vi "Start-Scope.vi"(0 "VISA resource name":refnum<visa-resource-name>="Scope", 1 "Vertical Range (10.0 V)":dbl=10.0, 3 "Position (0.0 s)":dbl, 4 "Acquisition Type (0:Sample)":u16(ring)=3 items=["Sample", "Peak Detect", "Hi Res", "Average", "Envelope", "WfmDB"], 5 "Signal Channel":u16(ring)=1 format="%#_5f" items=["Channel 1", "Channel 2", "Channel 3", "Channel 4", "Math 1", "Math 2", "Math 3", "Math 4", "Reference 1", "Reference 2", "Reference 3", "Reference 4"], 6 "Average Waveforms (10)":i32=300, 9 "Trigger Channel":u16(ring) format="%#_5f" items=["Channel 1", "Channel 2", "Channel 3", "Channel 4", "Math 1", "Math 2", "Math 3", "Math 4", "Reference 1", "Reference 2", "Reference 3", "Reference 4"], 11 "Input Impedance (0: 1M ohm)":u16(ring)=1 items=["1M", "50"], 12 "Record Length (10000)":u32=10000 caption="Record Length (10000s)", 13 "Trigger Level (0.0V)":dbl=1.0) -> (2 "Average Waveforms (10) Out":i32=300, 8 "error out":errorcluster, 10 "Timebase":u32, 14 "VISA resource name out":refnum<visa-resource-name>, 15 "Signal Channel \nOut":u16(ring)=1 caption="Signal Channel" format="%#_5f" items=["Channel 1", "Channel 2", "Channel 3", "Channel 4", "Math 1", "Math 2", "Math 3", "Math 4", "Reference 1", "Reference 2", "Reference 3", "Reference 4"])   [LabVIEW 2018]
uses:
  <instrlib>/Tektronix 7000 Series/Public/Configure/Configure Trigger (Edge).vi
  <instrlib>/Tektronix 7000 Series/Tektronix 7000 Series.lvlib
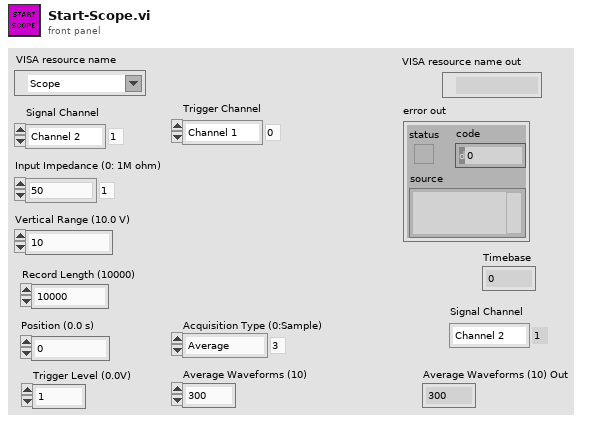
[diagram p1: front panel]
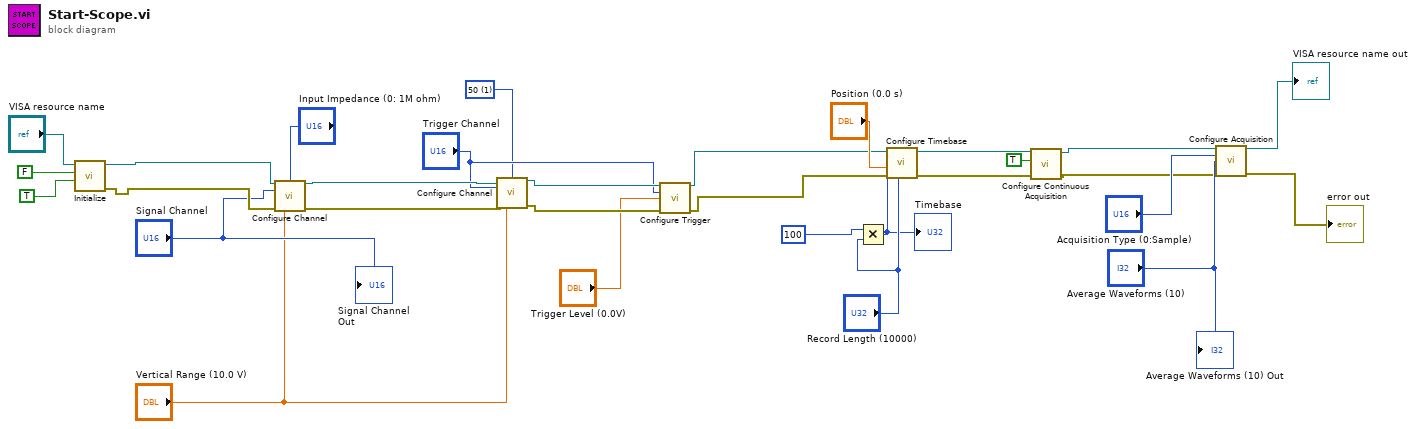
[diagram p0: block diagram]
diagram:
  w2 = u16 1 items=["1M", "50"] ("Input Impedance (0: 1M ohm)")
  n1 = call <instrlib>:"Initialize.vi"("Reset? ( Yes)"=TRUE, "ID Query? ( Yes)"=FALSE, "VISA resource name"="VISA resource name") -> ("error out"=w14:errorcluster, "VISA resource name out"=w15:refnum<visa-resource-name>)  [unwired: 7 in]
  n2 = call <instrlib>:"Configure Channel.vi"("VISA resource name"=w15, "Input Impedance (0: 1M ohm)"="Input Impedance (0: 1M ohm)", "Channel (0: Channel 1)"="Signal Channel", "error in (no error)"=w14, "Vertical Range (10.0 V)"="Vertical Range (10.0 V)") -> ("VISA resource name out"=w27:refnum<visa-resource-name>, "error out"=w26:errorcluster)  [unwired: 9 in]
  n3 = call <instrlib>:"Configure Channel.vi"("VISA resource name"=w27, "Input Impedance (0: 1M ohm)"=w2, "Channel (0: Channel 1)"="Trigger Channel", "error in (no error)"=w26, "Vertical Range (10.0 V)"="Vertical Range (10.0 V)") -> ("VISA resource name out"=w25:refnum<visa-resource-name>, "error out"=w24:errorcluster)  [unwired: 9 in]
  n4 = call-poly <instrlib>:"Configure Trigger.vi"("VISA resource name"=w25, "Source (0:Channel1)"="Trigger Channel", "Trigger Level (0.0V)"="Trigger Level (0.0V)", "error in (no error)"=w24) -> ("VISA resource name out"=w12:refnum<visa-resource-name>, "error out"=w11:errorcluster)  [unwired: 10 in]
  n5 = Multiply(x=u32 100, y="Record Length (10000)") -> (x*y=w18:u32)
  "Timebase" <- w18
  n6 = call <instrlib>:"Configure Timebase.vi"("Record Length (10000)"="Record Length (10000)", "error in (no error)"=w11, "Position (0.0 s)"="Position (0.0 s)", "Timebase (4 ns)"=w18, "VISA resource name"=w12) -> ("error out"=w9:errorcluster, "VISA resource name out"=w10:refnum<visa-resource-name>)  [unwired: 5 in]
  n7 = call <instrlib>:"Configure Continuous Acquisition.vi"("error in (no error)"=w9, "Enable Continuous Acquisition Mode (True)"=TRUE, "VISA resource name"=w10) -> ("error out"=w5:errorcluster, "VISA resource name out"=w6:refnum<visa-resource-name>)  [unwired: 7 in]
  n8 = call <instrlib>:"Configure Acquisition.vi"("VISA resource name"=w6, "Acquisition Type (0:Sample)"="Acquisition Type (0:Sample)", "Average Waveforms (10)"="Average Waveforms (10)", "error in (no error)"=w5) -> ("VISA resource name out"=→"VISA resource name out":refnum<visa-resource-name>, "error out"=→"error out":errorcluster)  [unwired: 10 in]
  "Signal Channel \nOut" <- "Signal Channel"
  "Average Waveforms (10) Out" <- "Average Waveforms (10)"
